vi "Send UpdateLinkCameraStatus.vi"(7 "Message Priority (Normal)":T2=enum."Normal", 8 "error in (no error)":errorcluster, 10 "LinkCameraStatus":T1=enum."Connected", 11 "Message Enqueuer":refnum<class "Message Enqueuer.lvclass">) -> (0 "error out":errorcluster, 3 "Message Enqueuer out":refnum<class "Message Enqueuer.lvclass">)   [LabVIEW 2020, in "ICameraTestingUI.lvlib" / "UpdateLinkCameraStatus Msg.lvclass"]
doc: "This VI sends the message to an actor."
uses:
  UpdateLinkCameraStatus Msg.lvclass
  UpdateLinkCameraStatus Msg.lvclass/UpdateLinkCameraStatus Msg.ctl
  <vilib>/ActorFramework/Message Enqueuer/Message Enqueuer.lvclass
  C:/Program Files (x86)/National Instruments/LabVIEW 2020/vi.lib/ActorFramework/Message/Message.lvclass
  <vilib>/ActorFramework/Message Enqueuer/Message Priority.ctl
  TypeDef/LinkCameraStatus.ctl
  TypeDef/ICameraTestingUI_typedef.lvlib
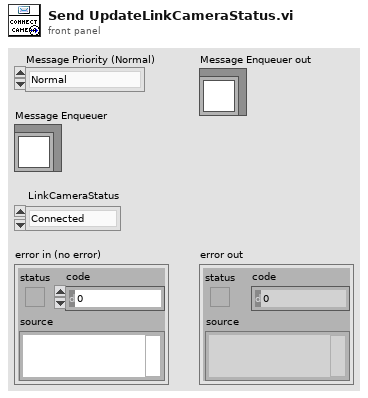
[diagram p1: front panel]
types:
  T1 = typedef "ICameraTestingUI_typedef.lvlib/LinkCameraStatus.ctl" = enum8{"Disconnected", "Connected", "Error"}
  T2 = typedef "Actor Framework.lvlib/Message Enqueuer.lvclass/Message Priority.ctl" = enum16{"Low", "Normal", "High"}
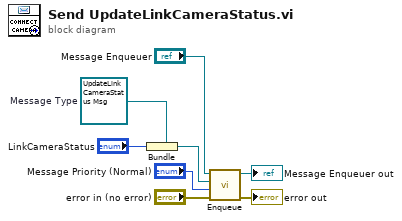
[diagram p0: block diagram]
diagram:
  w5 = refnum<class "UpdateLinkCameraStatus Msg.lvclass"> refnum  # Message Type
  n1 = Bundle(cluster=w5, "LinkCameraStatus") -> (w4:refnum<class "UpdateLinkCameraStatus Msg.lvclass">)
  n2 = call <vilib>:"Enqueue.vi"("error in (no error)"="error in (no error)", "Message Priority (Normal)"="Message Priority (Normal)", "Message"=w4, "Message Enqueuer in"="Message Enqueuer") -> ("error out"=→"error out":errorcluster, "Message Enqueuer out"=→"Message Enqueuer out":refnum<class "Message Enqueuer.lvclass">)  [unwired: 6 in]
